vi "D-Lockin.vi"(8 "error in (no error)":errorcluster, 9 "index":u32, 10 "Stop?":bool, 11 "SweepControl":refnum<class "SweepControl.lvclass">) -> (0 "error out":errorcluster, 3 "SweepControl":refnum<class "SweepControl.lvclass">)   [LabVIEW 2019, in "SweepControl.lvclass"]
uses:
  SweepControl.lvclass
  <userlib>/LevyLab/Lockin-Multichannel/Instrument.Lockin/Typedefs/Results Type--Enum.ctl
  SweepControl.lvclass/SweepControl.ctl
  Transport/Transport.lvclass/Transport.ctl
  Transport/Transport.lvclass
  Control Experiment/Control Experiment.lvclass
  <userlib>/LevyLab/Lockin-Multichannel/Instrument.Lockin/Instrument.Lockin.lvclass
panel:
  out "G4T":cluster{dbl[], dbl[]}[](graph)
  out "Y Lockins":cluster{dbl[], dbl[]}[](graph)
  out "X Lockins":cluster{dbl[], dbl[]}[](graph)
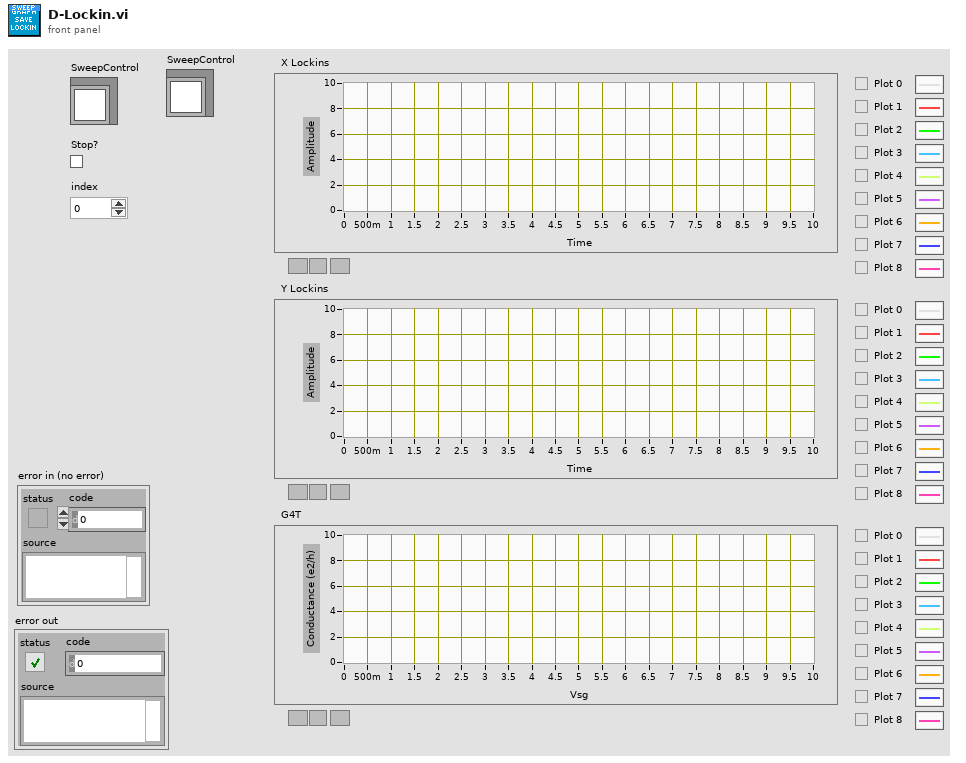
[diagram p1: front panel]
types:
  T1 = cluster{"Result X":dbl[], "Result Y":dbl[], "Data":cluster{"Y  Array":dbl[]}[], "wavenames":string[], "All Result X":dbl[][], "All Result Y":dbl[][]}
  T2 = cluster{"SweepControl":refnum<class "SweepControl.lvclass">, "data":cluster{"Result X":dbl[], "Result Y":dbl[], "Data":cluster{"Y  Array":dbl[]}[], "wavenames":string[], "All Result X":dbl[][], "All Result Y":dbl[][]}, "All Parameters":dbl[]}
  T3 = typedef "Instrument.Lockin.lvclass/Results Type--Enum.ctl" = enum16{"X", "Y", "R", "Theta", "Mean"}
  T4 = typedef "Control Experiment.lvclass/Instruments--cluster.ctl" = cluster{"KH7008":refnum<class "Instrument.KH7008.lvclass">[], "Lockin":refnum<class "Instrument.Lockin.lvclass">, "Temperature":refnum<class "Instrument.Cryostat.lvclass">, "Magnet":refnum<class "Instrument.Cryostat.lvclass">, "Rotator":refnum<class "Instrument.Cryostat.lvclass">, "Level":refnum<class "Instrument.Cryostat.lvclass">, "Capacitance Bridge":refnum<class "Instrument.CBridge.lvclass">, "Delay Line":refnum<class "Instrument.DelayLine.lvclass">, "Strain Cell":refnum<class "Instrument.Strain.lvclass">, "VNA":refnum<class "Instrument.VNA.lvclass">, "Voltage Source":refnum<class "Instrument.VSource.lvclass">}
  T5 = cluster{"I-":i32, "I+":i32, "V1-":i32, "V1+":i32, "I2-":i32, "I2+":i32, "V2-":i32, "V2+":i32}
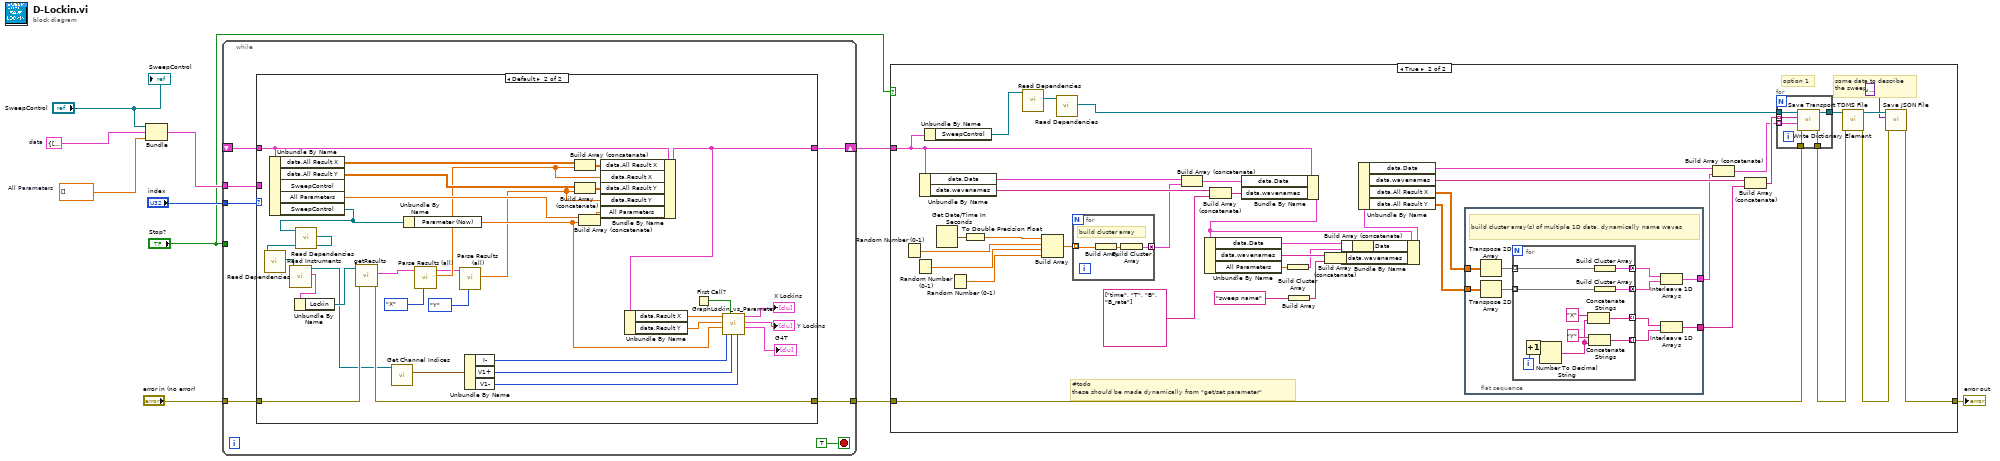
[diagram p0: block diagram]
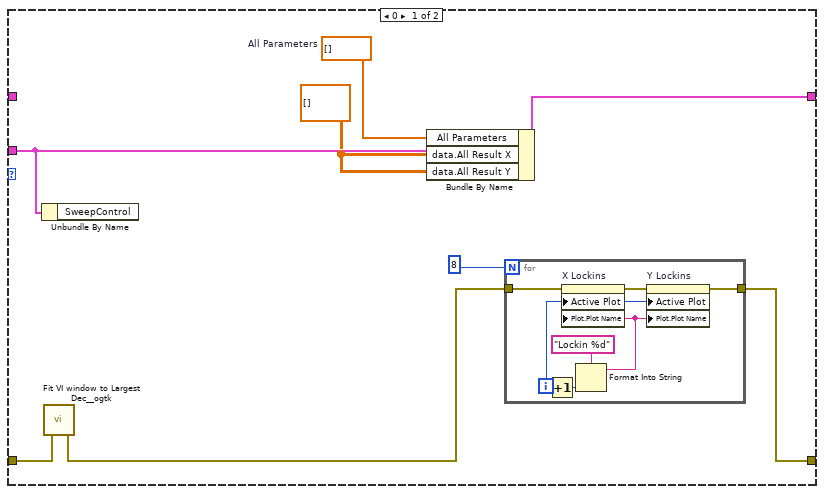
[diagram p3: hidden frame]
diagram:
  w3 = dbl[] []  # All Parameters
  w6 = T1 {"Result X"=[], "Result Y"=[], "Data"=[], "wavenames"=[], "All Result X"=[], "All Result Y"=[]}  # data
  n1 = Bundle("SweepControl"="SweepControl", "data"=w6, "All Parameters"=w3) -> (w7:T2)  [unwired: 1 in]
  n2 = while {
    tunnel: "index" -> [w17]
    tunnel: "Stop?" -> [_]
    tunnel: "error in (no error)" -> [w16]
    shift-right: [w14] -> w4
    shift-left: _ -> [w15]
    tunnel: w7 -> [w13]
    tunnel: [w12] -> w2
    stop <- TRUE stop-if-true
    n3 = case shown="Default" w17 {
      tunnel: w16 -> [w21 w61]
      tunnel: w15 -> [_ w59]
      tunnel: [w25 w57] -> w14
      tunnel: w13 -> [w24 _]
      tunnel: [w22 w60] -> w12
      frame 0 {
        w19 = dbl[] []  # All Parameters
        w20 = dbl[][] [] ("data.All Result X")
        n4 = Unbundle By Name(w24) -> ()  [unwired: 1 out]
        n5 = call <userlib>:"Fit VI window to Largest Dec__ogtk.vi"("error in (no error)"=w21) -> ("error out"=w18:errorcluster)  [unwired: 5 in, 1 out]
        n6 = Bundle By Name(cluster=w24, "All Parameters"=w19, "data.All Result X"=w20, "data.All Result Y"=w20) -> (w25:T2)
        n7 = for {
          N: 8 -> [_]
          tunnel: [w27] -> w22
          tunnel: w18 -> [w26]
          i -> [w30]
          n8 = Increment(x=w30) -> (x+1=w28:i32)
          n9 = Format Into String(format string="Lockin %d", w28) -> (resulting string=w31:string)  [unwired: 2 in, 1 out]
          n10 = property on="X Lockins" class="XYGraph (strict)"(error in=w26, "Active Plot"=w30, "Plot.Plot Name"=w31) -> (error out=w29:errorcluster)  [unwired: 1 in, 1 out]
          n11 = property on="Y Lockins" class="XYGraph (strict)"(error in=w29, "Active Plot"=w30, "Plot.Plot Name"=w31) -> (error out=w27:errorcluster)  [unwired: 1 in, 1 out]
        }
      }
      frame Default {
        n12 = Unbundle By Name(w59) -> ("data.All Result X"=w65:dbl[][], "data.All Result Y"=w64:dbl[][], "All Parameters"=w54:dbl[], "SweepControl"=w35:refnum<class "SweepControl.lvclass">)  [unwired: 1 out]
        n13 = call "Read Dependencies.vi"("SweepControl in"=w35) -> ("Transport"=w34:refnum<class "Transport.lvclass">)  [unwired: 8 in, 2 out]
        n14 = call "Read Dependencies.vi"("Transport"=w34) -> ("C.E."=w33:refnum<class "Control Experiment.lvclass">)  [unwired: 8 in, 2 out]
        n15 = call "Read Instruments.vi"("Control Experiment in"=w33) -> ("Instruments"=w48:T4, "Control Experiment out"=w46:refnum<class "Control Experiment.lvclass">)  [unwired: 8 in, 1 out]
        n16 = Unbundle By Name(w48) -> ("Lockin"=w47:refnum<class "Instrument.Lockin.lvclass">)
        n17 = call <userlib>:"getResults.vi"("error in (no error)"=w61, "Instrument.Lockin in"=w47) -> ("error out"=w60:errorcluster, "Results (Dictionary)"=w41:cluster{"key":string, "value":dbl}[])  [unwired: 6 in, 2 out]
        n18 = call "Get Channel Indices.vi"("Control Experiment in"=w46) -> ("Indices"=w45:T5)  [unwired: 8 in, 2 out]
        n19 = Unbundle By Name(w35) -> ("Parameter (Now)"=w53:dbl)
        n20 = call <userlib>:"Parse Results (all).vi"("Type"=Results_Type--Enum."X", "Results (Dictionary)"=w41) -> ("Data"=w40:dbl[], "Results (Dictionary)"=w38:cluster{"key":string, "value":dbl}[])  [unwired: 6 in, 2 out]
        n21 = call <userlib>:"Parse Results (all).vi"("Type"=Results_Type--Enum."Y", "Results (Dictionary)"=w38) -> ("Data"=w39:dbl[])  [unwired: 6 in, 3 out]
        n22 = Unbundle By Name(w45) -> ("I-"=w44:i32, "V1+"=w43:i32, "V1-"=w42:i32)
        n23 = Build Array (concatenate)(w65, w40) -> (w62:dbl[][])
        n24 = Build Array (concatenate)(w64, w39) -> (w63:dbl[][])
        n25 = Build Array (concatenate)(w54, w53) -> (w52:dbl[])
        n26 = Bundle By Name(cluster=w59, "data.All Result X"=w62, "data.Result X"=w40, "data.All Result Y"=w63, "data.Result Y"=w39, "All Parameters"=w52) -> (w57:T2)
        n27 = Unbundle By Name(w57) -> ("data.Result X"=w58:dbl[], "data.Result Y"=w55:dbl[])
        n28 = First Call?() -> (First Call?: T/F=w56:bool)
        n29 = call "GraphLockin_vs_Parameter.vi"("V-"=w42, "V+"=w43, "reset?"=w56, "Current"=w44, "Parameter"=w53, "Y[ ]"=w55, "X[ ]"=w58) -> ("G(e2/h) vs Parameter"=→"G4T":cluster{"Y":dbl[], "Y":dbl[]}[], "Y vs Parameter"=→"Y Lockins":cluster{dbl[], dbl[]}[], "X vs Parameter"=→"X Lockins":cluster{dbl[], dbl[]}[])  [unwired: 1 in, 1 out]
      }
    }
  }
  n30 = case shown="True" "Stop?" {
    tunnel: w4 -> [_ w81]
    tunnel: w2 -> [w66 w71]
    tunnel: [w66 w76] -> w1
    frame False {
    }
    frame True {
      # "option 1"
      # "some data to describe\nthe sweep"
      # "#todo\nthese should be made dynamically from \"get/set parameter\""
      n31 = Random Number (0-1)() -> (number: 0 to 1=w98:dbl)
      n32 = Random Number (0-1)() -> (number: 0 to 1=w97:dbl)
      n33 = Unbundle By Name(w81) -> ("data.Data"=w107:cluster{"Y  Array":dbl[]}[], "data.wavenames"=w106:string[])
      n34 = Unbundle By Name(w81) -> ("SweepControl"=w69:refnum<class "SweepControl.lvclass">)
      n35 = Get Date/Time In Seconds() -> (seconds since 1Jan1904=w102:timestamp)
      n36 = Random Number (0-1)() -> (number: 0 to 1=w96:dbl)
      n37 = To Double Precision Float(number=w102) -> (double precision float=w101:dbl)
      n38 = call "Read Dependencies.vi"("SweepControl in"=w69) -> ("Transport"=w68:refnum<class "Transport.lvclass">)  [unwired: 8 in, 2 out]
      n39 = Build Array(w101, w98, w97, w96) -> (w99:dbl[])
      n40 = call "Read Dependencies.vi"("Transport"=w68) -> ("C.E."=w67:refnum<class "Control Experiment.lvclass">)  [unwired: 8 in, 2 out]
      n41 = for {
        tunnel: [w136] -> w100 mode=concatenating
        tunnel: w99 -> [w135] mode=indexing
        # "build cluster array"
        n42 = Build Array(w135) -> (w137:dbl[])
        n43 = Build Cluster Array(w137) -> (w136:cluster{dbl[]}[])
      }
      n44 = Build Array (concatenate)(w107, w100) -> (w104:cluster{"Y  Array":dbl[]}[])
      n45 = Build Array (concatenate)(w106, string[] ["time", "T", "B", "B_rate"] ("wavenames (.Vx, etc)")) -> (w105:string[])
      n46 = Bundle By Name(cluster=w81, "data.Data"=w104, "data.wavenames"=w105) -> (w83:T2)
      n47 = Unbundle By Name(w83) -> ("data.Data"=w95:cluster{"Y  Array":dbl[]}[], "data.wavenames"=w94:string[], "All Parameters"=w92:dbl[])
      n48 = Build Cluster Array(w92) -> (w91:cluster{"All Parameters":dbl[]}[])
      n49 = Build Array("sweep name" ("wavenames")) -> (w88:string[])
      n50 = Build Array (concatenate)(w94, w88) -> (w90:string[])
      n51 = Build Array (concatenate)(w95, w91) -> (w93:cluster{"All Parameters":dbl[]}[])
      n52 = Bundle By Name(cluster=w83, "data.Data"=w93, "data.wavenames"=w90) -> (w82:T2)
      n53 = Unbundle By Name(w82) -> ("data.Data"=w87:cluster{"Y  Array":dbl[]}[], "data.wavenames"=w86:string[], "data.All Result X"=w85:dbl[][], "data.All Result Y"=w84:dbl[][])
      n54 = flat-sequence {
        tunnel: w85 -> [w123]
        tunnel: w84 -> [w122]
        tunnel: [w115] -> w80
        tunnel: [w114] -> w79
        frame #0 {
          # "build cluster array(s) of multiple 1D data, dynamically name waves"
          n55 = Transpose 2D Array(2D array=w123) -> (transposed array=w121:dbl[][])
          n56 = Transpose 2D Array(2D array=w122) -> (transposed array=w120:dbl[][])
          n57 = for {
            tunnel: w121 -> [w134] mode=indexing
            tunnel: w120 -> [w133] mode=indexing
            tunnel: [w132] -> w119 mode=concatenating
            tunnel: [w131] -> w118 mode=concatenating
            tunnel: [w126] -> w117 mode=indexing
            tunnel: [w125] -> w116 mode=indexing
            i -> [w128]
            n58 = Increment(x=w128) -> (x+1=w124:i32)
            n59 = Number To Decimal String(number=w124) -> (decimal integer string=w127:string)  [unwired: 1 in]
            n60 = Concatenate Strings("X" ("wavenames"), w127) -> (w126:string)
            n61 = Concatenate Strings("Y" ("wavenames"), w127) -> (w125:string)
            n62 = Build Cluster Array(w134) -> (w132:cluster{dbl[]}[])
            n63 = Build Cluster Array(w133) -> (w131:cluster{dbl[]}[])
          }
          n64 = Interleave 1D Arrays(w119, w118) -> (w114:cluster{dbl[]}[])
          n65 = Interleave 1D Arrays(w117, w116) -> (w115:string[])
        }
      }
      n66 = Build Array (concatenate)(w87, w79) -> (w72:cluster{"Y  Array":dbl[]}[])
      n67 = Build Array (concatenate)(w86, w80) -> (w73:string[])
      n68 = for {
        tunnel: [w113] -> w74
        tunnel: w73 -> [w112] mode=indexing
        tunnel: w72 -> [w111] mode=indexing
        tunnel: w67 -> [w110]
        tunnel: w71 -> [w109]
        tunnel: [w108] -> w70
        n69 = call "Write Dictionary Element.vi"("error in (no error)"=w109, "value"=w111, "key"=w112, "Control Experiment in"=w110) -> ("error out"=w108:errorcluster, "Control Experiment out"=w113:refnum<class "Control Experiment.lvclass">)  [unwired: 6 in]
      }
      n70 = call "Save Transport TDMS File.vi"("error in (no error)"=w70, "Control Experiment in"=w74) -> ("error out"=w78:errorcluster, "Control Experiment out"=w77:refnum<class "Control Experiment.lvclass">)  [unwired: 8 in]
      n71 = call "Save JSON File.vi"("error in (no error)"=w78, "Data"=variant, "Control Experiment in"=w77) -> ("error out"=w76:errorcluster)  [unwired: 8 in]
    }
  }
  "error out" <- w1
  "SweepControl" <- "SweepControl"
